vi "CLSUIP_GetNonGrowableHeight.vi"(8 "error in (no error)":errorcluster, 10 "Number of growable terminals":i32, 11 "Growable Node Ref":refnum<vi>) -> (0 "error out":errorcluster, 2 "Non-Growable height":i32, 3 "Growable Node Ref out":refnum<vi>)   [LabVIEW 2021, in "MemberVICreation.lvlib"]
uses:
  <resource>/Framework/Providers/LVClassLibrary/NewAccessors/MemberVICreation.lvlib
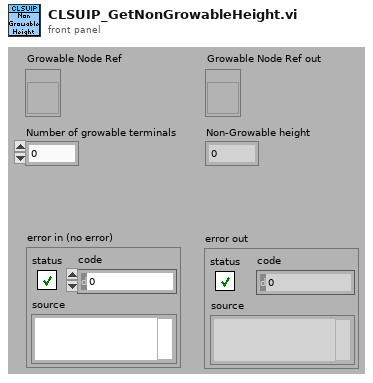
[diagram p1: front panel]
types:
  T1 = typedef "LVRectTypeDef.ctl" = cluster{"left":i16, "top":i16, "right":i16, "bottom":i16}
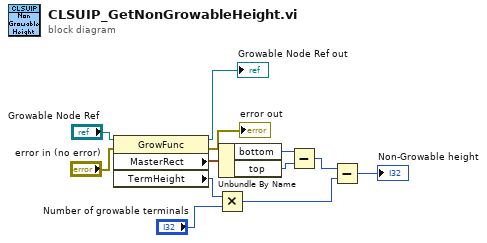
[diagram p0: block diagram]
diagram:
  n1 = property class="GrowFunc"(reference="Growable Node Ref", error in="error in (no error)") -> (reference out=→"Growable Node Ref out":refnum<vi>, error out=→"error out":errorcluster, "MasterRect"=w9:T1, "TermHeight"=w6:i32)
  n2 = Multiply(x=w6, y="Number of growable terminals") -> (x*y=w3:i32)
  n3 = Unbundle By Name(w9) -> ("bottom"=w8:i16, "top"=w7:i16)
  n4 = Subtract(x=w8, y=w7) -> (x-y=w4:i16)
  n5 = Subtract(x=w4, y=w3) -> (x-y=→"Non-Growable height":i32)
